vi "TAF_amp.vi"(0 "Counters In":u32[](array[numeric]), 1 "Counter Rng":T3(array[cluster]), 2 "AmpClust":T1 {"AmpMode" items=["Below Hits", "Above Hits"]}, 3 "Freq Values":dbl[](array[numeric]), 5 "Templates":dbl[][](array[numeric]) format="%#_2g", 7 "Amp Array":i16[](array[numeric]), 9 "In Data":i16[](array[numeric]), 13 "FreqClust":T2 {"FreqMode" items=["Below Hits", "Above Hits", "Between Hits", "Outside Hits"]}, 14 "Thresholds":dbl[](array[numeric]) format="%.2f") -> (4 "LeftOverAmp":i16[](array[numeric]), 6 "Left Over":i16[](array[numeric]), 8 "Array":dbl[](array[numeric]) format="%.2f", 10 "Counters Out":u32[](array[numeric]), 11 "Targ Syll Freq":dbl, 12 "NoteDetect":bool, 15 "Trigger":bool)   [LabVIEW 2018]
uses:
  <vilib>/Analysis/NI_AALPro.lvlib
  <vilib>/Analysis/4window.llb/Hamming Window (DBL).vi
  <vilib>/Analysis/2dsp.llb/Power Spectrum (DBL).vi
panel:
  out "AmpFFT":dbl[](array[numeric])
  out "MinF":i32
  out "MaxV":i32
  out "fft error":i32
  out "Power Spec Size":i32[](array[numeric])
  in  "Input Power Spec":dbl[][](array[numeric])
  out "Left Over Size":i32
  out "Nfftu":i32
  # "OR"
  # "AND"
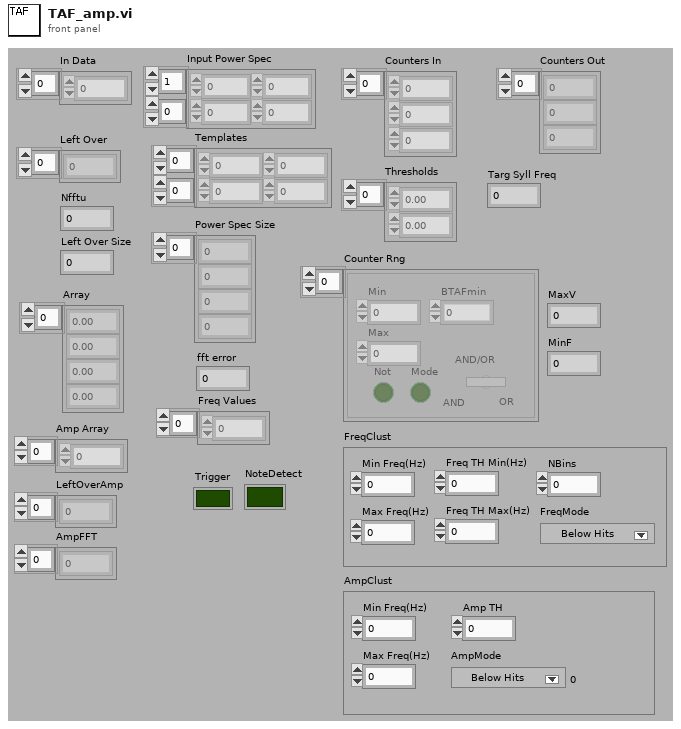
[diagram p1: front panel]
types:
  T1 = cluster{"Min Freq(Hz)":dbl, "Max Freq(Hz)":dbl, "Amp TH":dbl, "AmpMode":u16}
  T2 = cluster{"Min Freq(Hz)":dbl, "Max Freq(Hz)":dbl, "Freq TH Min(Hz)":dbl, "Freq TH Max(Hz)":dbl, "NBins":i32, "FreqMode":u16}
  T3 = cluster{"Min":i16, "Max":i16, "Not":bool, "Mode":bool, "BTAFmin":i16, "AND/OR":bool}[]
  T4 = cluster{"Min":i16, "Max":i16, "Not":bool, "Mode":bool, "BTAFmin":i16, "AND/OR":bool}
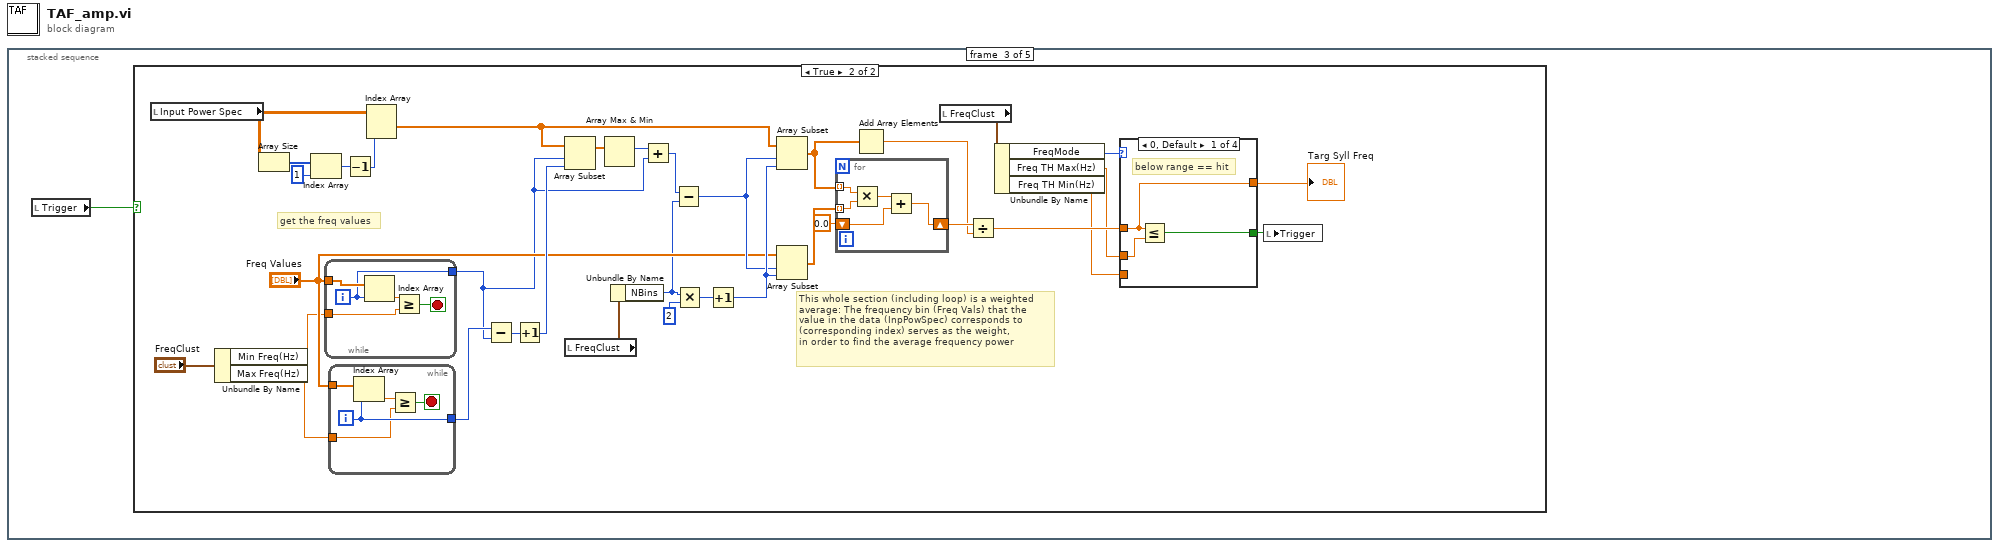
[diagram p0: block diagram]
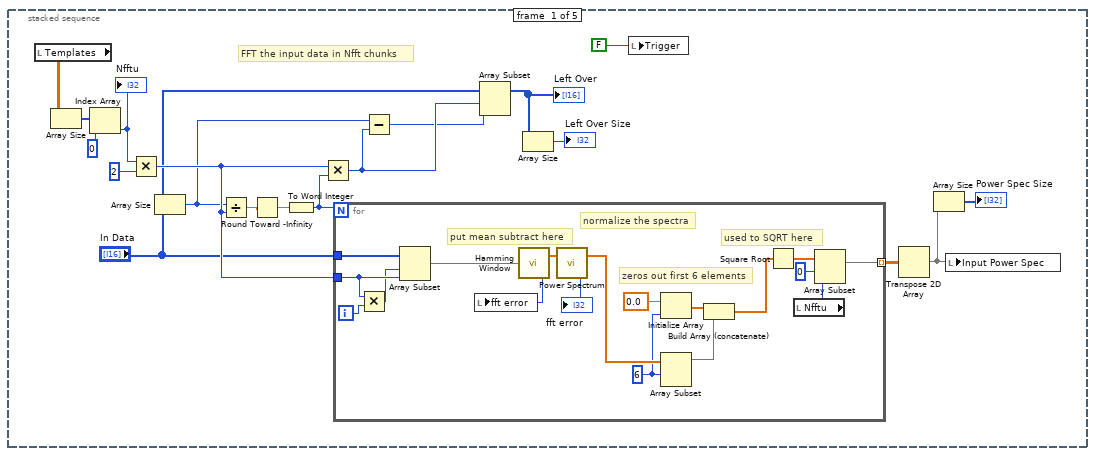
[diagram p2: hidden frame]
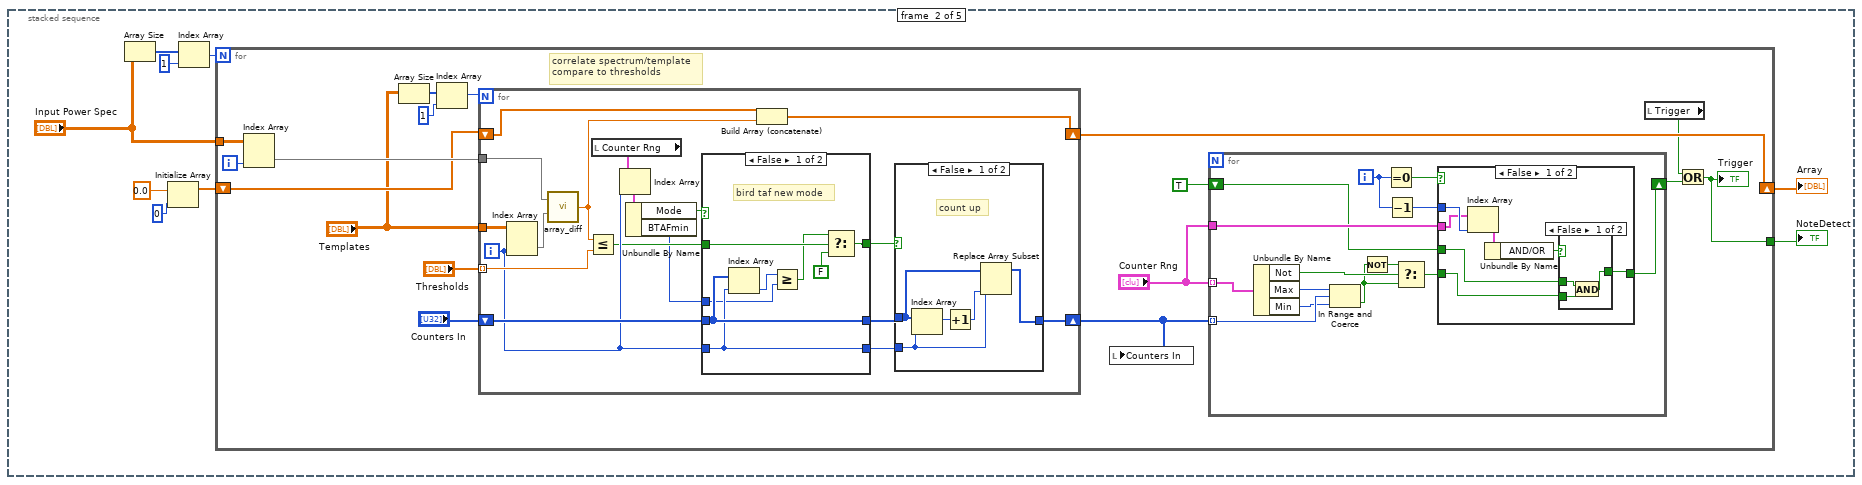
[diagram p3: hidden frame]
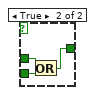
[diagram p4: hidden frame]
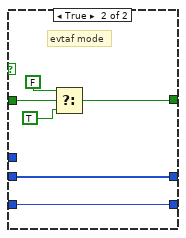
[diagram p6: hidden frame]
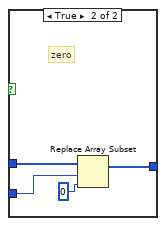
[diagram p7: hidden frame]
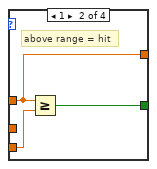
[diagram p9: hidden frame]
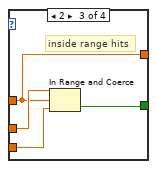
[diagram p10: hidden frame]
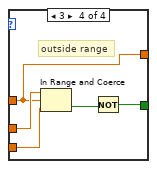
[diagram p11: hidden frame]
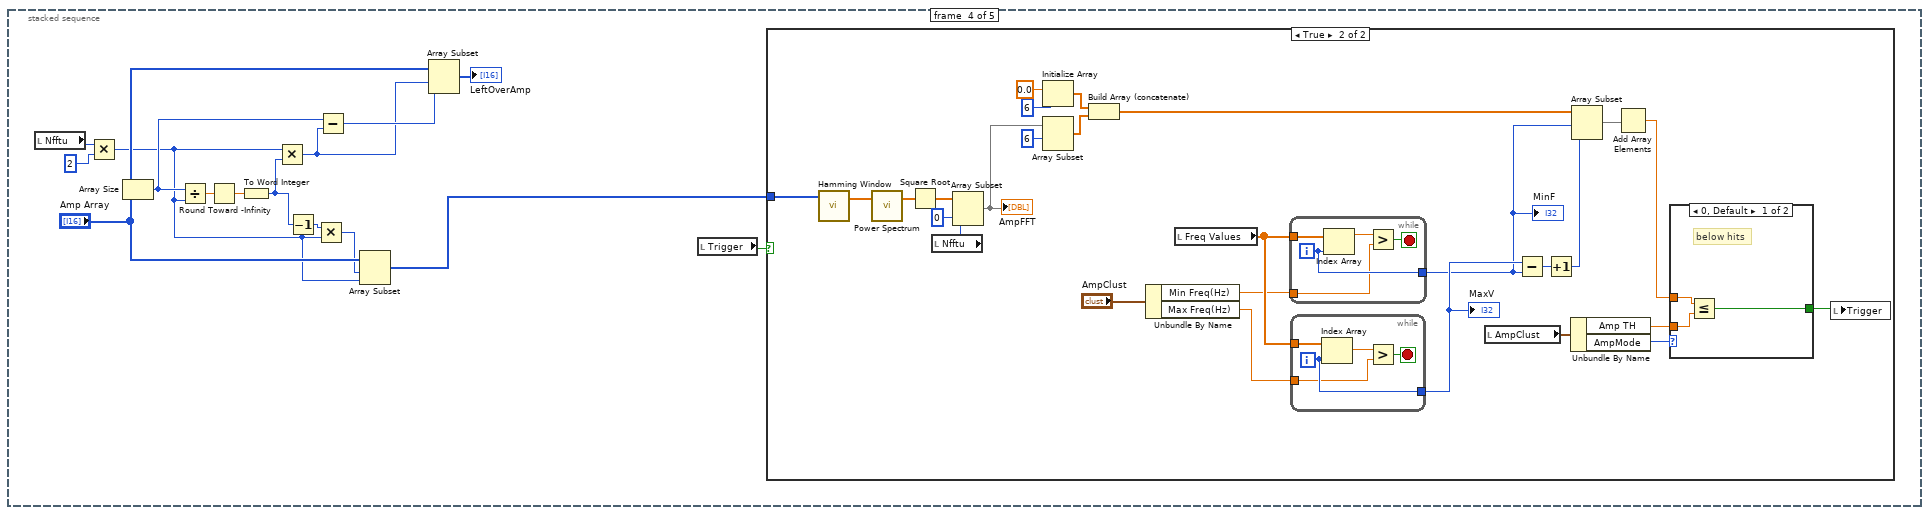
[diagram p12: hidden frame]
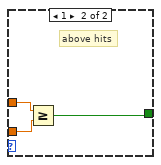
[diagram p14: hidden frame]
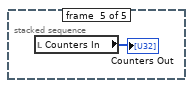
[diagram p15: hidden frame]
diagram:
  n1 = stacked-sequence {
    frame #0 {
      # "FFT the input data in Nfft chunks"
      n2 = local read "Templates"() -> (w15:dbl[][])
      n3 = Array Size(array=w15) -> (size(s)=w14:i32[])
      n4 = Index Array(array=w14, index=0 ("Index")) -> (element=w5:i32)
      "Nfftu" <- w5
      n5 = Multiply(x=w5, y=2) -> (x*y=w12:i32)
      n6 = Array Size(array="In Data") -> (size(s)=w9:i32)
      n7 = Divide(x=w9, y=w12) -> (x/y=w19:dbl)
      n8 = Round Toward -Infinity(1:w19) -> (0:w18:dbl)
      n9 = To Word Integer(number=w18) -> (16bit integer=w10:i16)
      n10 = Multiply(x=w12, y=w10) -> (x*y=w17:i32)
      n11 = for {
        N: w10 -> [_]
        tunnel: "In Data" -> [w37]
        tunnel: w12 -> [w35]
        tunnel: [w26] -> w8 mode=indexing
        i -> [w36]
        w22 = 6 ("Array Index")
        # "used to SQRT here"
        # "zeros out first 6 elements"
        # "put mean subtract here"
        # "normalize the spectra"
        n12 = Multiply(x=w35, y=w36) -> (x*y=w34:i32)
        n13 = Array Subset(array=w37, index=w34, length=w35) -> (w25:i16[])
        n14 = call-poly <vilib>:"Hamming Window.vi"("X"=w25) -> ("Windowed X"=w32:dbl[], "error"=w33:i32)
        n15 = local write "fft error"(w33) -> ()
        n16 = call-poly <vilib>:"Power Spectrum.vi"("X"=w32) -> ("Power Spectrum"=w30:dbl[], "error"=→"fft error":i32)
        n17 = Initialize Array(0.0 ("Element Data"), w22) -> (w28:dbl[])
        n18 = Array Subset(array=w30, index=w22) -> (w27:dbl[])  [unwired: 1 in]
        n19 = Build Array (concatenate)(w28, w27) -> (w21:dbl[])
        n20 = Square Root(x=w21) -> (sqrt(x)=w20:dbl[])
        n21 = local read "Nfftu"() -> (w24:i32)
        n22 = Array Subset(array=w20, index=0 ("Array Index"), length=w24) -> (w26:dbl[])
      }
      n23 = Subtract(x=w9, y=w17) -> (x-y=w16:i32)
      n24 = Array Subset(array="In Data", index=w17, length=w16) -> (w6:i16[])
      "Left Over" <- w6
      n25 = Array Size(array=w6) -> (size(s)=→"Left Over Size":i32)
      n26 = local write "Trigger"(FALSE ("Trigger")) -> ()
      n27 = Transpose 2D Array(2D array=w8) -> (transposed array=w3:dbl[][])
      n28 = Array Size(array=w3) -> (size(s)=→"Power Spec Size":i32[])
      n29 = local write "Input Power Spec"(w3) -> ()
    }
    frame #1 {
      n30 = Array Size(array="Input Power Spec") -> (size(s)=w46:i32[])
      n31 = Initialize Array(0.0 ("Element Data"), 0 ("Dimension Size")) -> (w41:dbl[])
      n32 = Index Array(array=w46, index=1 ("Index")) -> (element=w44:i32)
      n33 = for {
        N: w44 -> [_]
        tunnel: "Input Power Spec" -> [w63]
        shift-right: [w56] -> w40
        shift-left: w41 -> [w57]
        tunnel: [w49] -> w38
        i -> [w62]
        # "correlate spectrum/template\ncompare to thresholds"
        n34 = Index Array(array=w63, index (col)=w62) -> (element=w58:dbl[])  [unwired: 1 in]
        n35 = Array Size(array="Templates") -> (size(s)=w59:i32[])
        n36 = Index Array(array=w59, index=1 ("Index")) -> (element=w61:i32)
        n37 = for {
          N: w61 -> [_]
          tunnel: w58 -> [w108]
          tunnel: "Templates" -> [w107]
          tunnel: "Thresholds" -> [w106] mode=indexing
          shift-right: [w105] -> w52
          shift-left: "Counters In" -> [w99]
          shift-right: [w101] -> w56
          shift-left: w57 -> [w103]
          i -> [w98]
          n38 = Index Array(array=w107, index (col)=w98) -> (element=w109:dbl[])  [unwired: 1 in]
          n39 = call "array_diff.vi"("Normalized Template"=w109, "In"=w108) -> ("Out"=w102:dbl)
          n40 = Less Or Equal?(x=w102, y=w106) -> (x <= y?=w94:bool)
          n41 = local read "Counter Rng"() -> (w100:T3)
          n42 = Index Array(array=w100, index=w98) -> (element=w104:T4)
          n43 = Unbundle By Name(w104) -> ("Mode"=w95:bool, "BTAFmin"=w92:i16)
          n44 = case shown="False" w95 {
            tunnel: w99 -> [w117 w123]
            tunnel: w98 -> [w116 w122]
            tunnel: [w117 w123] -> w97
            tunnel: [w116 w122] -> w96
            tunnel: w94 -> [w113 w121]
            tunnel: [w110 w118] -> w93
            tunnel: w92 -> [w114 _]
            frame False {
              # "bird taf new mode"
              n45 = Index Array(array=w117, index=w116) -> (element=w115:u32)
              n46 = Greater Or Equal?(x=w115, y=w114) -> (x >= y?=w111:bool)
              n47 = Select(t=w111, s=w113, f=FALSE) -> (s? t:f=w110:bool)
            }
            frame True {
              # "evtaf mode"
              n48 = Select(t=FALSE, s=w121, f=TRUE) -> (s? t:f=w118:bool)
            }
          }
          n49 = Build Array (concatenate)(w103, w102) -> (w101:dbl[])
          n50 = case shown="False" w93 {
            tunnel: w97 -> [w125 w132]
            tunnel: w96 -> [w126 w130]
            tunnel: [w124 w129] -> w105
            frame False {
              # "count up"
              n51 = Index Array(array=w125, index=w126) -> (element=w128:u32)
              n52 = Increment(x=w128) -> (x+1=w127:u32)
              n53 = Replace Array Subset(array=w125, new element=w127, index=w126) -> (w124:u32[])
            }
            frame True {
              # "zero"
              n54 = Replace Array Subset(array=w132, new element=u32 0 ("Element Data"), index=w130) -> (w129:u32[])
            }
          }
        }
        n55 = local write "Counters In"(w52) -> ()
        n56 = for {
          tunnel: "Counter Rng" -> [w76] mode=indexing
          tunnel: w52 -> [w77] mode=indexing
          shift-right: [w68] -> w47
          shift-left: TRUE -> [w64]
          tunnel: "Counter Rng" -> [w67]
          i -> [w66]
          n57 = Unbundle By Name(w76) -> ("Not"=w73:bool, "Max"=w75:i16, "Min"=w74:i16)
          n58 = In Range and Coerce(upper limit=w75, x=w77, lower limit=w74) -> (In Range?=w71:bool)  [unwired: 1 out]
          n59 = Not(x=w71) -> (.not. x?=w72:bool)
          n60 = Equal To 0?(x=w66) -> (x = 0?=w70:bool)
          n61 = Decrement(x=w66) -> (x-1=w65:i32)
          n62 = Select(t=w72, s=w73, f=w71) -> (s? t:f=w69:bool)
          n63 = case shown="False" w70 {
            tunnel: w69 -> [w80 w91]
            tunnel: [w78 w91] -> w68
            tunnel: w67 -> [w83 _]
            tunnel: w65 -> [w84 _]
            tunnel: w64 -> [w79 _]
            frame False {
              n64 = Index Array(array=w83, index=w84) -> (element=w82:T4)
              n65 = Unbundle By Name(w82) -> ("AND/OR"=w81:bool)
              n66 = case shown="False" w81 {
                tunnel: w80 -> [w86 w89]
                tunnel: w79 -> [w87 w90]
                tunnel: [w85 w88] -> w78
                frame False {
                  n67 = And(x=w87, y=w86) -> (x .and. y?=w85:bool)
                }
                frame True {
                  n68 = Or(x=w90, y=w89) -> (x .or. y?=w88:bool)
                }
              }
            }
            frame True {
            }
          }
        }
        n69 = local read "Trigger"() -> (w51:bool)
        n70 = Or(x=w51, y=w47) -> (x .or. y?=w49:bool)
        "Trigger" <- w49
      }
      "Array" <- w40
      "NoteDetect" <- w38
    }
    frame #2 {
      n71 = local read "Trigger"() -> (w133:bool)
      n72 = case shown="True" w133 {
        frame False {
        }
        frame True {
          # "This whole section (including loop) is a weighted\naverage: The frequency bin (Freq Vals) that the \nvalue in the data (InpPowSpec) corresponds to\n(corresponding index) serves as the weight,\nin order to find the average frequency power"
          # "get the freq values"
          n73 = local read "Input Power Spec"() -> (w140:dbl[][])
          n74 = Unbundle By Name("FreqClust") -> ("Min Freq(Hz)"=w146:dbl, "Max Freq(Hz)"=w145:dbl)
          n75 = Array Size(array=w140) -> (size(s)=w139:i32[])
          n76 = Index Array(array=w139, index=1) -> (element=w137:i32)
          n77 = while {
            tunnel: "Freq Values" -> [w183]
            tunnel: [w180] -> w151
            tunnel: w146 -> [w179]
            i -> [w180]
            stop <- w181 stop-if-true
            n78 = Index Array(array=w183, index=w180) -> (element=w182:dbl)
            n79 = Greater Or Equal?(x=w182, y=w179) -> (x >= y?=w181:bool)
          }
          n80 = while {
            tunnel: "Freq Values" -> [w178]
            tunnel: [w175] -> w165
            tunnel: w145 -> [w174]
            i -> [w175]
            stop <- w176 stop-if-true
            n81 = Index Array(array=w178, index=w175) -> (element=w177:dbl)
            n82 = Greater Or Equal?(x=w177, y=w174) -> (x >= y?=w176:bool)
          }
          n83 = Decrement(x=w137) -> (x-1=w136:i32)
          n84 = Index Array(array=w140, index (col)=w136) -> (element=w135:dbl[])  [unwired: 1 in]
          n85 = Subtract(x=w165, y=w151) -> (x-y=w168:i32)
          n86 = Increment(x=w168) -> (x+1=w167:i32)
          n87 = Array Subset(array=w135, index=w151, length=w167) -> (w164:dbl[])
          n88 = local read "FreqClust"() -> (w144:T2)
          n89 = Array Max & Min(array=w164) -> (max index (indices)=w152:i32)  [unwired: 3 out]
          n90 = Unbundle By Name(w144) -> ("NBins"=w143:i32)
          n91 = Add(x=w152, y=w151) -> (x+y=w150:i32)
          n92 = Subtract(x=w150, y=w143) -> (x-y=w160:i32)
          n93 = Multiply(x=w143, y=2) -> (x*y=w162:i32)
          n94 = Increment(x=w162) -> (x+1=w161:i32)
          n95 = Array Subset(array=w135, index=w160, length=w161) -> (w157:dbl[])
          n96 = Array Subset(array="Freq Values", index=w160, length=w161) -> (w159:dbl[])
          n97 = for {
            tunnel: w157 -> [w173] mode=indexing
            tunnel: w159 -> [w172] mode=indexing
            shift-right: [w169] -> w156
            shift-left: 0.0 -> [w170]
            n98 = Multiply(x=w173, y=w172) -> (x*y=w171:dbl)
            n99 = Add(x=w171, y=w170) -> (x+y=w169:dbl)
          }
          n100 = Add Array Elements(numeric array=w157) -> (sum=w155:dbl)
          n101 = local read "FreqClust"() -> (w149:T2)
          n102 = Divide(x=w156, y=w155) -> (x/y=w154:dbl)
          n103 = Unbundle By Name(w149) -> ("FreqMode"=w148:u16, "Freq TH Max(Hz)"=w141:dbl, "Freq TH Min(Hz)"=w142:dbl)
          n104 = case shown="0, Default" w148 {
            tunnel: w141 -> [w186 _ w193 w198]
            tunnel: [w185 w189 w191 w195] -> w166
            tunnel: w154 -> [w184 w187 w190 w194]
            tunnel: w142 -> [_ w188 w192 w197]
            tunnel: [w184 w187 w190 w194] -> w134
            frame 0, Default {
              # "below range == hit"
              n105 = Less Or Equal?(x=w184, y=w186) -> (x <= y?=w185:bool)
            }
            frame 1 {
              # "above range = hit"
              n106 = Greater Or Equal?(x=w187, y=w188) -> (x >= y?=w189:bool)
            }
            frame 2 {
              # "inside range hits"
              n107 = In Range and Coerce(upper limit=w193, x=w190, lower limit=w192) -> (In Range?=w191:bool)  [unwired: 1 out]
            }
            frame 3 {
              # "outside range"
              n108 = In Range and Coerce(upper limit=w198, x=w194, lower limit=w197) -> (In Range?=w196:bool)  [unwired: 1 out]
              n109 = Not(x=w196) -> (.not. x?=w195:bool)
            }
          }
          "Targ Syll Freq" <- w134
          n110 = local write "Trigger"(w166) -> ()
        }
      }
    }
    frame #3 {
      n111 = local read "Nfftu"() -> (w212:i32)
      n112 = Multiply(x=w212, y=2) -> (x*y=w200:i32)
      n113 = Array Size(array="Amp Array") -> (size(s)=w208:i32)
      n114 = Divide(x=w208, y=w200) -> (x/y=w210:dbl)
      n115 = Round Toward -Infinity(1:w210) -> (0:w209:dbl)
      n116 = To Word Integer(number=w209) -> (16bit integer=w204:i16)
      n117 = Multiply(x=w200, y=w204) -> (x*y=w206:i32)
      n118 = Decrement(x=w204) -> (x-1=w203:i16)
      n119 = Multiply(x=w203, y=w200) -> (x*y=w201:i32)
      n120 = Subtract(x=w208, y=w206) -> (x-y=w207:i32)
      n121 = Array Subset(array="Amp Array", index=w201, length=w200) -> (w199:i16[])
      n122 = Array Subset(array="Amp Array", index=w206, length=w207) -> (→"LeftOverAmp":i16[])
      n123 = local read "Trigger"() -> (w213:bool)
      n124 = case shown="True" w213 {
        tunnel: w199 -> [_ w221]
        frame False {
        }
        frame True {
          n125 = call-poly <vilib>:"Hamming Window.vi"("X"=w221) -> ("Windowed X"=w222:dbl[])  [unwired: 1 out]
          n126 = call-poly <vilib>:"Power Spectrum.vi"("X"=w222) -> ("Power Spectrum"=w223:dbl[])  [unwired: 1 out]
          n127 = Square Root(x=w223) -> (sqrt(x)=w224:dbl[])
          n128 = local read "Nfftu"() -> (w226:i32)
          n129 = Array Subset(array=w224, index=0, length=w226) -> (w218:dbl[])
          "AmpFFT" <- w218
          n130 = Initialize Array(0.0 ("element"), 6 ("dimension size")) -> (w220:dbl[])
          n131 = Array Subset(array=w218, index=6) -> (w219:dbl[])  [unwired: 1 in]
          n132 = Build Array (concatenate)(w220, w219) -> (w214:dbl[])
          n133 = Unbundle By Name("AmpClust") -> ("Min Freq(Hz)"=w238:dbl, "Max Freq(Hz)"=w237:dbl)
          n134 = local read "Freq Values"() -> (w240:dbl[])
          n135 = while {
            tunnel: w240 -> [w256]
            tunnel: [w255] -> w234
            tunnel: w238 -> [w253]
            i -> [w255]
            stop <- w252 stop-if-true
            n136 = Index Array(array=w256, index=w255) -> (element=w254:dbl)
            n137 = Greater?(x=w254, y=w253) -> (0:w252:bool)
          }
          "MinF" <- w234
          n138 = while {
            tunnel: w240 -> [w251]
            tunnel: [w250] -> w236
            tunnel: w237 -> [w249]
            i -> [w250]
            stop <- w247 stop-if-true
            n139 = Index Array(array=w251, index=w250) -> (element=w248:dbl)
            n140 = Greater?(x=w248, y=w249) -> (0:w247:bool)
          }
          "MaxV" <- w236
          n141 = local read "AmpClust"() -> (w230:T1)
          n142 = Subtract(x=w236, y=w234) -> (x-y=w235:i32)
          n143 = Increment(x=w235) -> (x+1=w233:i32)
          n144 = Unbundle By Name(w230) -> ("Amp TH"=w228:dbl, "AmpMode"=w229:u16)
          n145 = Array Subset(array=w214, index=w234, length=w233) -> (w232:dbl[])
          n146 = Add Array Elements(numeric array=w232) -> (sum=w231:dbl)
          n147 = case shown="0, Default" w229 {
            tunnel: w231 -> [w243 w246]
            tunnel: w228 -> [w242 w245]
            tunnel: [w241 w244] -> w227
            frame 0, Default {
              # "below hits"
              n148 = Less Or Equal?(x=w243, y=w242) -> (x <= y?=w241:bool)
            }
            frame 1 {
              # "above hits"
              n149 = Greater Or Equal?(x=w246, y=w245) -> (x >= y?=w244:bool)
            }
          }
          n150 = local write "Trigger"(w227) -> ()
        }
      }
    }
    frame #4 {
      n151 = local read "Counters In"() -> (→"Counters Out":u32[])
    }
  }
